vi "Debug Write String.vi"(6 "include timestamp? (F)":bool, 7 "prefix (\"\")":string, 8 "error in (no error)":errorcluster, 9 "clear before next write (F)":bool, 11 "value":string) -> (0 "error out":errorcluster)   [LabVIEW 2020, in "Debug Log.lvlib"]
doc: "This VI has the same behavior as Debug Write VI when wired with a string. This VI is not a VI macro, so it is useful for debugging complex G situations where higher level operations of G are not allowed (such as debugging XNodes themselves)."
uses:
  <vilib>/Utility/Debug Log/Debug Log.lvlib
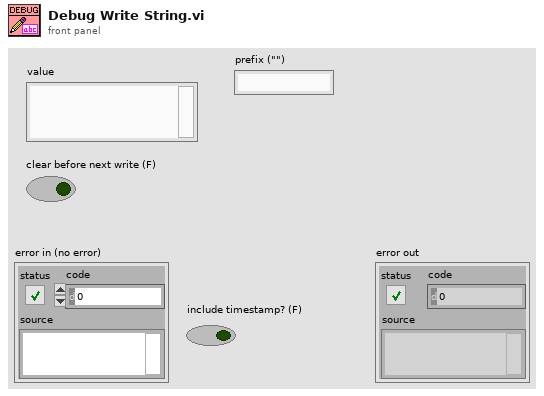
[diagram p1: front panel]
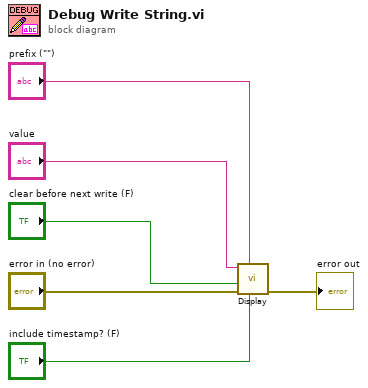
[diagram p0: block diagram]
diagram:
  n1 = call <vilib>:"Display.vi"("include timestamp? (F)"="include timestamp? (F)", "prefix (\"\")"="prefix (\"\")", "error in (no error)"="error in (no error)", "clear before next write (F)"="clear before next write (F)", "log text"="value") -> ("error out"=→"error out":errorcluster)  [unwired: 6 in]
